vi "Set HW Interface Digital Outputs.vi"(8 "error in (no error)":errorcluster, 10 "Digital Outputs":T1, 11 "Hardware Interface in":refnum<class "Hardware Interface.lvclass">) -> (0 "error out":errorcluster, 3 "Hardware Interface out":refnum<class "Hardware Interface.lvclass">)   [LabVIEW 2013, in "Hardware Interface.lvclass"]
uses:
  Hardware Interface.lvclass
  BoolArrayWithName.ctl
  Hardware Interface.lvclass/Hardware Interface.ctl
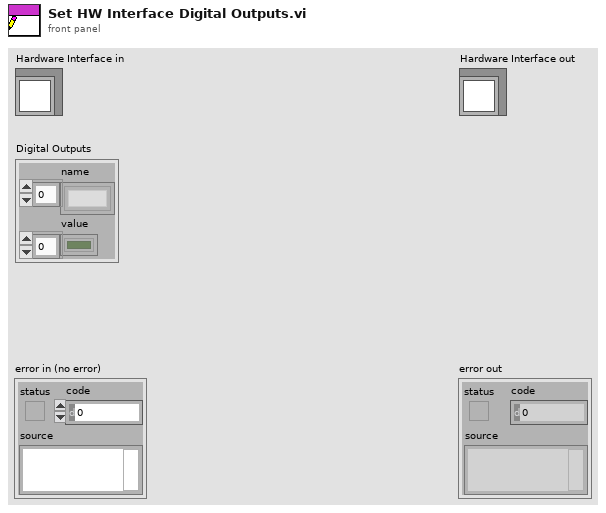
[diagram p1: front panel]
types:
  T1 = typedef "Hardware Interface.lvclass/BoolArrayWithName.ctl" = cluster{"name":string[], "value":bool[]}
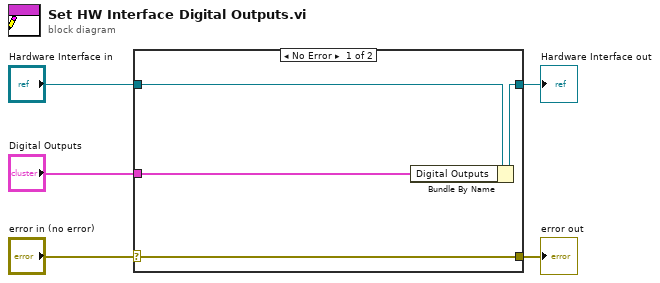
[diagram p0: block diagram]
diagram:
  n1 = case shown="No Error" "error in (no error)" {
    selector: "error in (no error)" -> [w9 w10]
    tunnel: [w9 w10] -> w4
    tunnel: [w7 w11] -> w2
    tunnel: "Hardware Interface in" -> [w8 w11]
    tunnel: "Digital Outputs" -> [w6 _]
    frame No Error {
      n2 = Bundle By Name(cluster=w8, "Digital Outputs"=w6) -> (w7:refnum<class "Hardware Interface.lvclass">)
    }
    frame Error {
    }
  }
  "error out" <- w4
  "Hardware Interface out" <- w2
